vi "Durability_will_2012_12_10_main.vi"() -> ()   [LabVIEW 2011]
uses:
  Program Files/National Instruments/LabVIEW 2011/resource/objmgr/daqmx.rc
panel:
  out "error out":errorcluster
  in  "Speed 2/3":i8(slide)=100 min=0 max=100 step=10 scale=0.0..100.0
  in  "Speed 1":i8(slide)=50 min=0 max=100 step=10 scale=0.0..100.0
  in  "Motor 3":bool
  in  "Motor 2":bool
  in  "Motor 1":bool=TRUE
  in  "Quit 4":bool
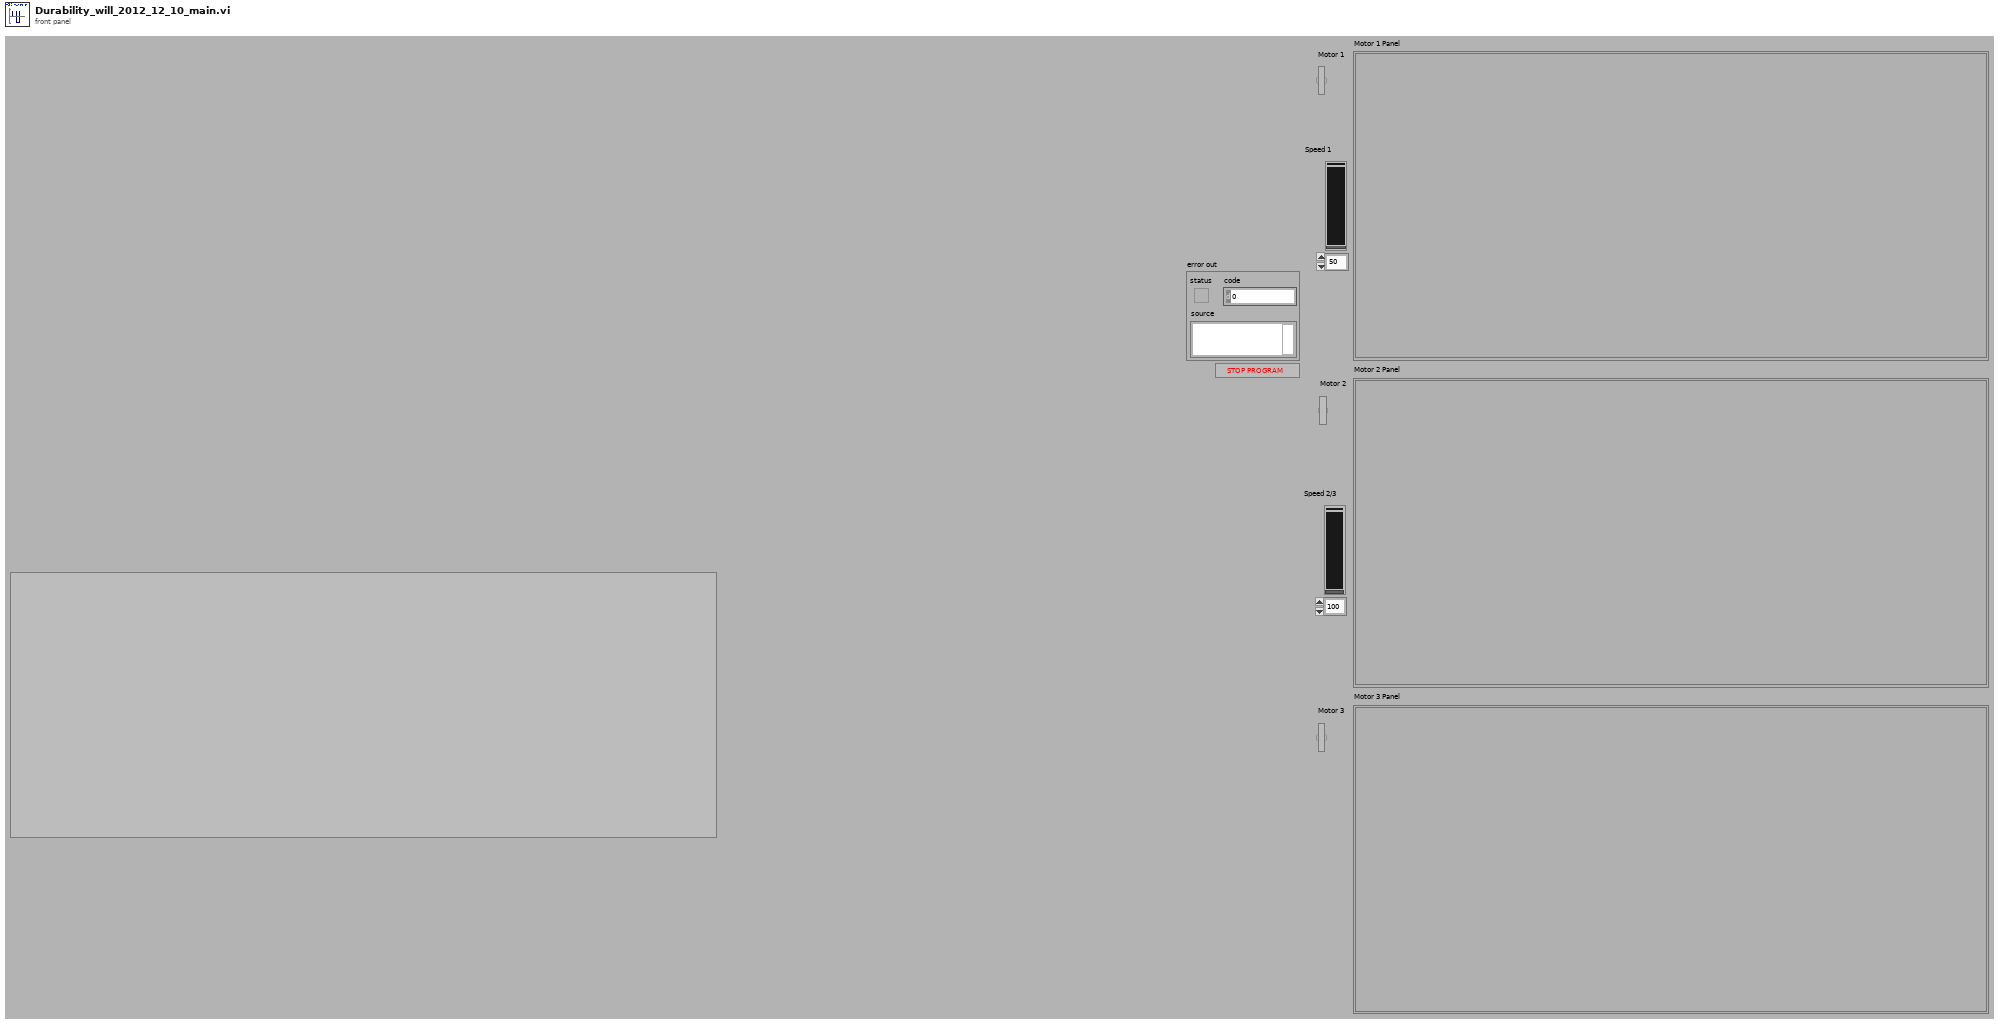
[diagram p1: front panel]
types:
  T1 = enum8{"Enabled", "Disabled", "Disabled and Grayed Out"}
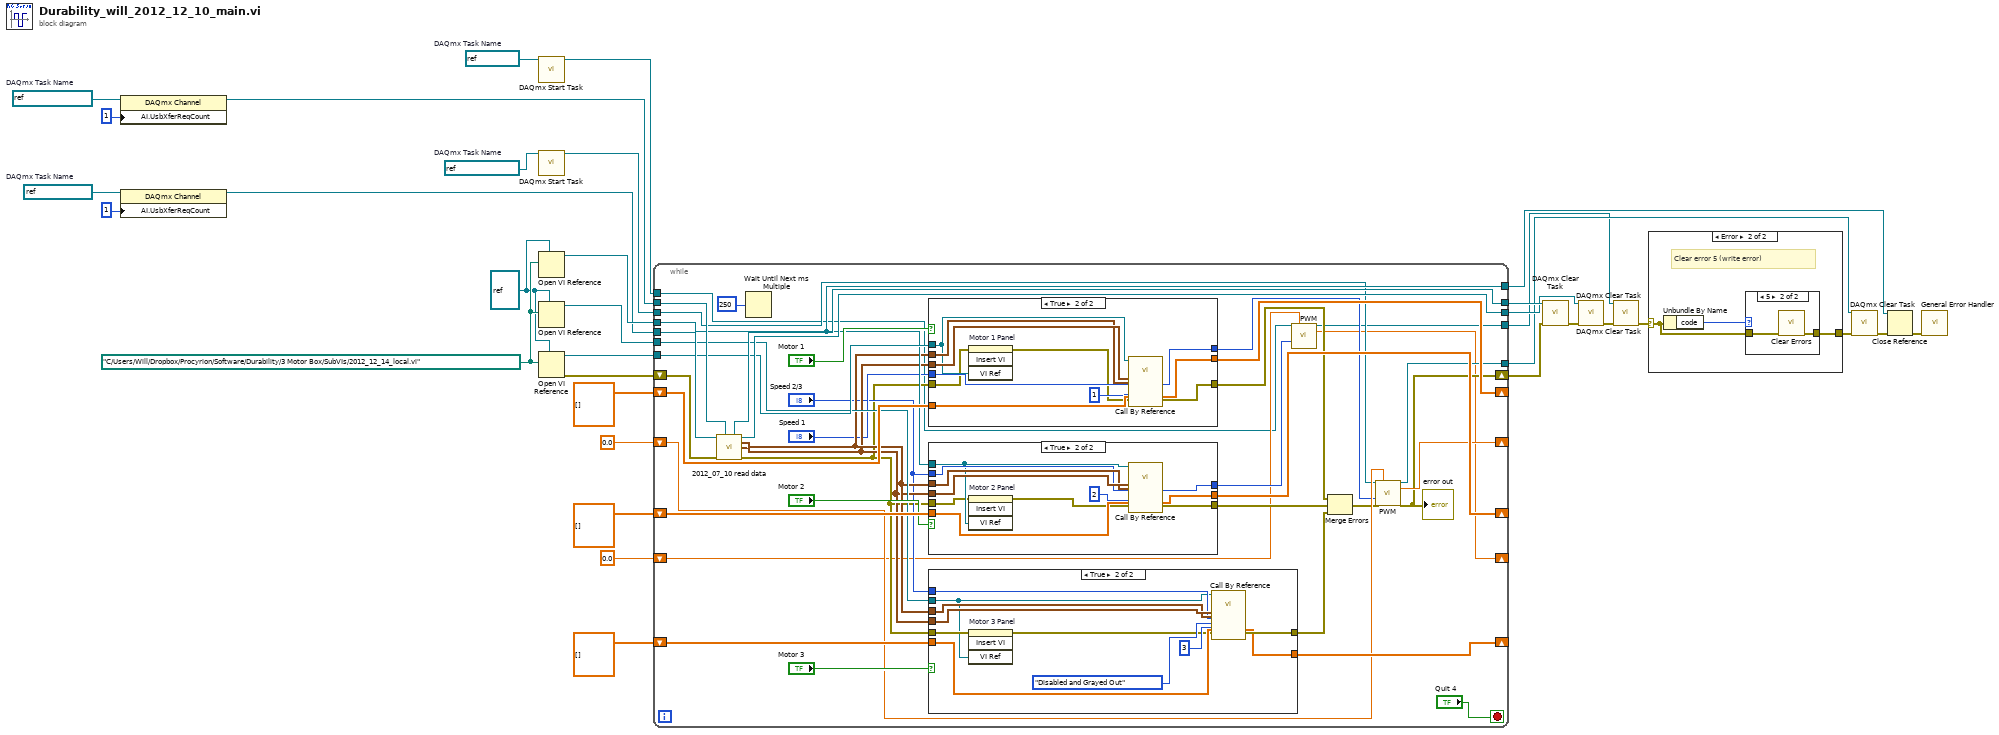
[diagram p0: block diagram]
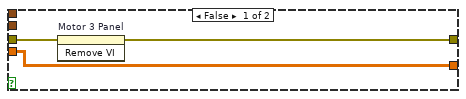
[diagram p4: hidden frame]
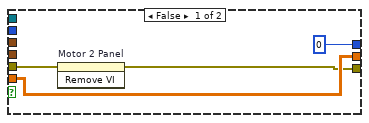
[diagram p5: hidden frame]
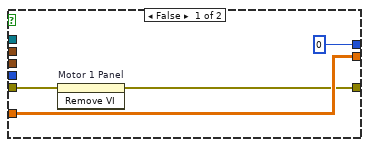
[diagram p6: hidden frame]
diagram:
  w5 = refnum<k21> "PWM 2"  # DAQmx Task Name
  w18 = path "C:/Users/Will/Dropbox/Procyrion/Software/Durability/3 Motor Box/SubVIs/2012_12_14_local.vi" ("'each motor' path")
  w17 = refnum<vi> refnum ("type specifier VI Refnum (for type only)")
  w21 = refnum<k21> "PWM Signal"  # DAQmx Task Name
  w11 = refnum<k21> "MC Power"  # DAQmx Task Name
  w7 = refnum<k21> "Motor Power"  # DAQmx Task Name
  n1 = property class="DAQmx Channel"(reference=w7, "AI.UsbXferReqCount"=u32 1) -> (reference out=w6:refnum<k21>)  [unwired: 1 in, 1 out]
  n2 = property class="DAQmx Channel"(reference=w11, "AI.UsbXferReqCount"=u32 1) -> (reference out=w10:refnum<k21>)  [unwired: 1 in, 1 out]
  n3 = call <vilib>:"DAQmx Start Task.vi"("task/channels in"=w5) -> ("task out"=w4:refnum<k21>)  [unwired: 13 in, 1 out]
  n4 = call <vilib>:"DAQmx Start Task.vi"("task/channels in"=w21) -> ("task out"=w19:refnum<k21>)  [unwired: 13 in, 1 out]
  n5 = Open VI Reference(type specifier VI Refnum (for type only)=w17, vi path=w18) -> (vi reference=w13:refnum<vi>)  [unwired: 4 in, 1 out]
  n6 = Open VI Reference(type specifier VI Refnum (for type only)=w17, vi path=w18) -> (vi reference=w12:refnum<vi>)  [unwired: 4 in, 1 out]
  n7 = Open VI Reference(type specifier VI Refnum (for type only)=w17, vi path=w18) -> (vi reference=w14:refnum<vi>, error out=w20:errorcluster)  [unwired: 4 in]
  n8 = while {
    tunnel: w10 -> [w70]
    tunnel: w6 -> [w69]
    shift-right: [w65] -> _
    shift-left: dbl[][][] [] -> [w66]
    shift-right: [w42] -> w33
    shift-left: w20 -> [w58]
    shift-right: [w47] -> _
    shift-left: 0.0 -> [w48]
    tunnel: [w68] -> w28
    tunnel: [w67] -> w27
    shift-right: [w62] -> _
    shift-left: dbl[][][] [] -> [w63]
    shift-right: [w38] -> _
    shift-left: 0.0 -> [w36]
    tunnel: w14 -> [w61]
    tunnel: [w59] -> w24
    tunnel: w13 -> [w59]
    tunnel: w19 -> [w39]
    shift-right: [w57] -> _
    shift-left: dbl[][][] [] -> [w56]
    tunnel: w12 -> [w55]
    tunnel: [w51] -> w16
    tunnel: w4 -> [w35]
    tunnel: [w34] -> w3
    stop <- "Quit 4" stop-if-true
    n9 = call "2012_07_10 read data.vi"("MC Power"=w70, "Motor Power"=w69, "Error In"=w58) -> ("Motor Power Out"=w68:refnum<k21>, "MC Power Out"=w67:refnum<k21>, "Motor Power Data"=w53:waveform(dbl)[], "MC Power Data"=w52:waveform(dbl)[], "error out"=w45:errorcluster)  [unwired: 8 in]
    n10 = Wait Until Next ms Multiple(millisecond multiple=u32 250) -> ()  [unwired: 1 out]
    n11 = case shown="True" "Motor 1" {
      tunnel: [w103 w111] -> w40
      tunnel: w45 -> [w102 w107]
      tunnel: w66 -> [w105 w115]
      tunnel: [w105 w116] -> w65
      tunnel: w52 -> [_ w113]
      tunnel: w53 -> [_ w112]
      tunnel: w61 -> [_ w108]
      tunnel: "Speed 1" -> [_ w110]
      tunnel: [i8 0 ("Power \nSetting") w109] -> w46
      frame False {
        n12 = invoke on="Motor 1 Panel" class="SubPnl" method="Remove VI"(error in=w102) -> (error out=w103:errorcluster)  [unwired: 2 in, 2 out]
      }
      frame True {
        n13 = invoke on="Motor 1 Panel" class="SubPnl" method="Insert VI"(error in=w107, "VI Ref"=w108) -> (error out=w106:errorcluster)  [unwired: 2 in, 3 out]
        n14 = call-by-ref "?"(reference=w108, "MC Power Data In"=w113, "Motor Power Data In"=w112, "Power \nSetting"=w110, "Motor"=i16 1, "Error In"=w106, "Fine Data In"=w115) -> ("Power \nSetting"=w109:i8, "Fine Data Out"=w116:dbl[][][], "Errors"=w111:errorcluster)  [unwired: 8 in, 2 out]
      }
    }
    n15 = case shown="True" "Motor 2" {
      tunnel: [w88 w101] -> w41
      tunnel: w63 -> [w90 w99]
      tunnel: [w90 w100] -> w62
      tunnel: w59 -> [_ w93]
      tunnel: w52 -> [_ w97]
      tunnel: w53 -> [_ w96]
      tunnel: w45 -> [w87 w92]
      tunnel: "Speed 2/3" -> [_ w95]
      tunnel: [i8 0 ("Power \nSetting") w94] -> w37
      frame False {
        n16 = invoke on="Motor 2 Panel" class="SubPnl" method="Remove VI"(error in=w87) -> (error out=w88:errorcluster)  [unwired: 2 in, 2 out]
      }
      frame True {
        n17 = invoke on="Motor 2 Panel" class="SubPnl" method="Insert VI"(error in=w92, "VI Ref"=w93) -> (error out=w91:errorcluster)  [unwired: 2 in, 3 out]
        n18 = call-by-ref "?"(reference=w93, "MC Power Data In"=w97, "Motor Power Data In"=w96, "Power \nSetting"=w95, "Motor"=i16 2, "Error In"=w91, "Fine Data In"=w99) -> ("Power \nSetting"=w94:i8, "Fine Data Out"=w100:dbl[][][], "Errors"=w101:errorcluster)  [unwired: 8 in, 2 out]
      }
    }
    n19 = case shown="True" "Motor 3" {
      tunnel: [w73 w86] -> w44
      tunnel: w56 -> [w75 w84]
      tunnel: [w75 w85] -> w57
      tunnel: w55 -> [_ w76]
      tunnel: w52 -> [_ w82]
      tunnel: w53 -> [_ w81]
      tunnel: w45 -> [w74 w78]
      tunnel: "Speed 2/3" -> [_ w80]
      frame False {
        n20 = invoke on="Motor 3 Panel" class="SubPnl" method="Remove VI"(error in=w74) -> (error out=w73:errorcluster)  [unwired: 2 in, 2 out]
      }
      frame True {
        n21 = invoke on="Motor 3 Panel" class="SubPnl" method="Insert VI"(error in=w78, "VI Ref"=w76) -> (error out=w77:errorcluster)  [unwired: 2 in, 3 out]
        n22 = call-by-ref "?"(reference=w76, "MC Power Data In"=w82, "Motor Power Data In"=w81, "Power \nSetting"=w80, "On/Off Control"=T1."Disabled and Grayed Out", "Motor"=i16 3, "Error In"=w77, "Fine Data In"=w84) -> ("Fine Data Out"=w85:dbl[][][], "Errors"=w86:errorcluster)  [unwired: 7 in, 3 out]
      }
    }
    n23 = call "PWM.vi"("Refnum in"=w35, "Speed 1"=w37, "High Time In 1"=w36) -> ("Refnum out"=w34:refnum<k21>, "High Time Out 1"=w38:dbl)  [unwired: 22 in, 1 out]
    n24 = Merge Errors(w40, w41, w44) -> (w43:errorcluster)
    n25 = call "PWM.vi"("Refnum in"=w39, "Speed 1"=w46, "error in (no error)"=w43, "High Time In 1"=w48) -> ("Refnum out"=w51:refnum<k21>, "High Time Out 1"=w47:dbl, "error out"=w42:errorcluster)  [unwired: 21 in]
    "error out" <- w42
  }
  n26 = call <vilib>:"DAQmx Clear Task.vi"("task in"=w28, "error in"=w33) -> ("error out"=w30:errorcluster)  [unwired: 13 in]
  n27 = call <vilib>:"DAQmx Clear Task.vi"("task in"=w27, "error in"=w30) -> ("error out"=w2:errorcluster)  [unwired: 13 in]
  n28 = call <vilib>:"DAQmx Clear Task.vi"("task in"=w3, "error in"=w2) -> ("error out"=w1:errorcluster)  [unwired: 13 in]
  n29 = case shown="Error" w1 {
    selector: w1 -> [w117 w119]
    tunnel: [w117 w118] -> w31
    frame No Error {
    }
    frame Error {
      # "Clear error 5 (write error)"
      n30 = Unbundle By Name(w119) -> ("code"=w120:i32)
      n31 = case shown="5" w120 {
        tunnel: w119 -> [w121 w123]
        tunnel: [w121 w122] -> w118
        frame Default {
        }
        frame 5 {
          n32 = call <vilib>:"Clear Errors.vi"("error in (no error)"=w123) -> ("error out"=w122:errorcluster)  [unwired: 6 in]
        }
      }
    }
  }
  n33 = call <vilib>:"DAQmx Clear Task.vi"("task in"=w16, "error in"=w31) -> ("error out"=w23:errorcluster)  [unwired: 13 in]
  n34 = Close Reference(reference=w24, error in (no error)=w23) -> (error out=w22:errorcluster)
  n35 = call <vilib>:"General Error Handler.vi"("error in (no error)"=w22) -> ()  [unwired: 10 in, 5 out]
